vi "add.vi"(1 "b":dbl, 2 "a":dbl) -> (0 "result":dbl)   [LabVIEW 2019]
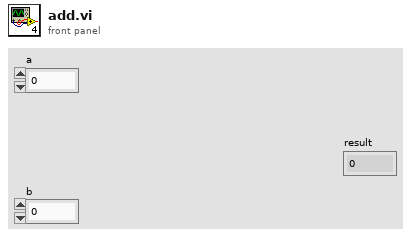
[diagram p1: front panel]
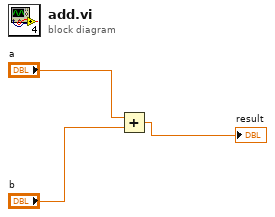
[diagram p0: block diagram]
diagram:
  n1 = Add(x="a", y="b") -> (x+y=→"result":dbl)
